vi "WPI_AnalogChannelGetAverageVoltageNavX.vi"(8 "error in":errorcluster, 11 "AIDeviceRef":T1={"DevStatus"={"status"=FALSE, "code"=0, "source"=""}, "Analog Channel"=enum."AI 1"}) -> (0 "error out":errorcluster, 2 "Voltage":dbl, 3 "AIDeviceRef":T1={"DevStatus"={"status"=FALSE, "code"=0, "source"=""}, "Analog Channel"=enum."AI 1"})   [LabVIEW 2025]
doc: "Returns the average voltage value from the oversample and average engine for the channel. The converter scales the raw value to the voltage value using the least significant bit weight constant and the offset constant of the hardware. Oversampling increases the resolution of the voltage value but decreases the update rate. Averaging returns a stable voltage value but also decreases the update rate. Use the GetVoltage VI to get voltage values directly from the A/D converter.\n\nThis software is licensed. Open the labview\\readme\\WPI Robotics Library Open Source License.txt file for more information."
uses:
  <vilib>/Rock Robotics/WPI/AnalogChannel/WPI_AnalogChannelDevRef.ctl
  <vilib>/Rock Robotics/SystemInterfaces/AI/FPGA_AIChannel.ctl
  <vilib>/ptbypt/NI_PtbyPt.lvlib
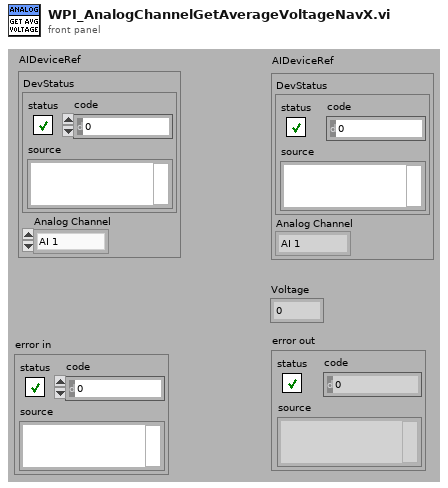
[diagram p1: front panel]
types:
  T1 = typedef "WPI_AnalogChannelDevRef.ctl" = cluster{"DevStatus":errorcluster, "Analog Channel":T2}
  T2 = typedef "FPGA_AIChannel.ctl" = enum8{"AI 0", "AI 1", "AI 2", "AI 3", "AI MXP 0", "AI MXP 1", "AI MXP 2", "AI MXP 3", "Invalid"}
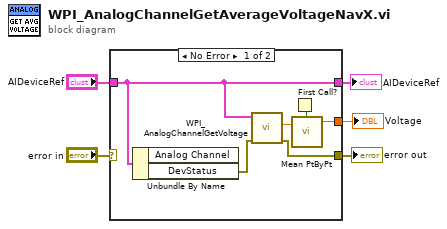
[diagram p0: block diagram]
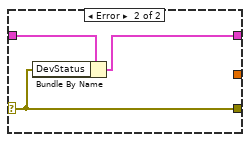
[diagram p2: hidden frame]
diagram:
  n1 = case shown="No Error" "error in" {
    selector: "error in" -> [_ w12]
    tunnel: "AIDeviceRef" -> [w6 w14]
    tunnel: [w6 w13] -> w4
    tunnel: [w9 _] -> w3
    tunnel: [w10 w12] -> w1
    frame No Error {
      n2 = Unbundle By Name(w6) -> ("DevStatus"=w11:errorcluster)  [unwired: 1 out]
      n3 = call <vilib>:"WPI_AnalogChannelGetVoltage.vi"("error in (no error)"=w11, "AIDeviceRef"=w6) -> ("error out"=w10:errorcluster, "Voltage"=w8:dbl)  [unwired: 7 in, 1 out]
      n4 = First Call?() -> (First Call?: T/F=w7:bool)
      n5 = call <vilib>:"Mean PtByPt.vi"("x"=w8, "initialize"=w7) -> ("mean"=w9:dbl)  [unwired: 2 in, 1 out]
    }
    frame Error {
      n6 = Bundle By Name(cluster=w14, "DevStatus"=w12) -> (w13:T1)
    }
  }
  "AIDeviceRef" <- w4
  "Voltage" <- w3
  "error out" <- w1
